vi "Write SubPanelReference.vi"(8 "error in (no error)":errorcluster, 10 "SubPanelReference":refnum<vi>, 11 "EmbeddedSMO in":refnum<class "Embedded UI.lvclass">) -> (0 "error out":errorcluster, 3 "EmbeddedSMO out":refnum<class "Embedded UI.lvclass">)   [LabVIEW 2019, in "Embedded UI.lvclass"]
uses:
  Embedded UI.lvclass
  Embedded UI.lvclass/Embedded UI.ctl
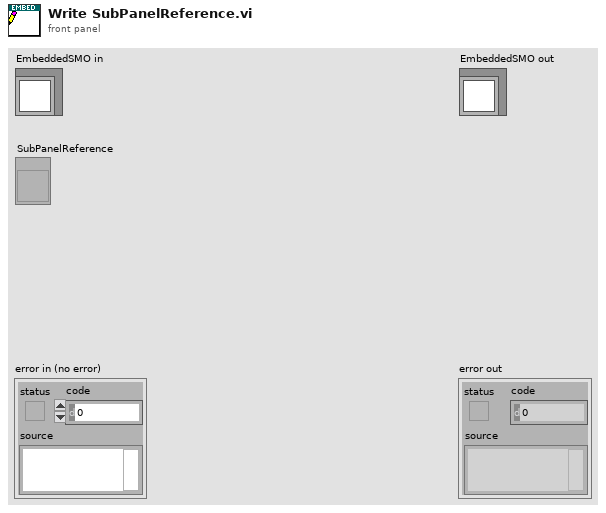
[diagram p1: front panel]
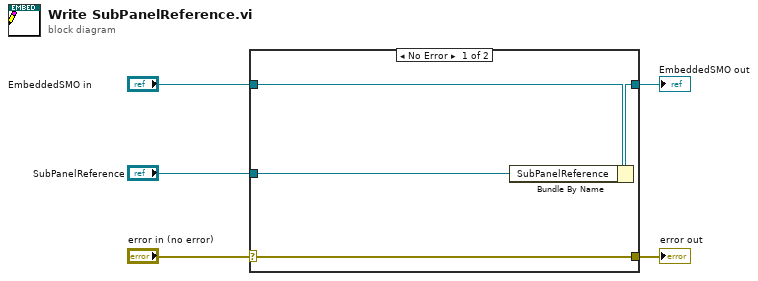
[diagram p0: block diagram]
diagram:
  n1 = case shown="No Error" "error in (no error)" {
    selector: "error in (no error)" -> [w9 w10]
    tunnel: [w9 w10] -> w4
    tunnel: [w7 w11] -> w2
    tunnel: "EmbeddedSMO in" -> [w8 w11]
    tunnel: "SubPanelReference" -> [w6 _]
    frame No Error {
      n2 = Bundle By Name(cluster=w8, "SubPanelReference"=w6) -> (w7:refnum<class "Embedded UI.lvclass">)
    }
    frame Error {
    }
  }
  "error out" <- w4
  "EmbeddedSMO out" <- w2
